vi "Write Receiver.vi"(10 "Receiver":string, 11 "Debug Data In":refnum<class "Debug Data.lvclass">) -> (3 "Debug Data Out":refnum<class "Debug Data.lvclass">)   [LabVIEW 2020, in "Debug Data.lvclass"]
uses:
  Debug Data.lvclass
  Debug Data.lvclass/Debug Data.ctl
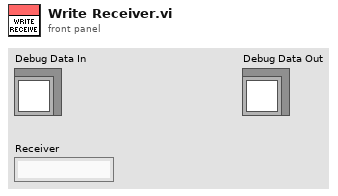
[diagram p1: front panel]
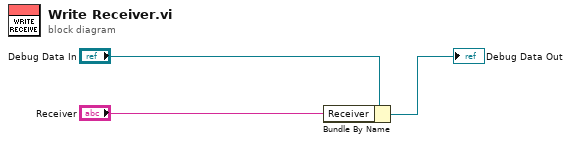
[diagram p0: block diagram]
diagram:
  n1 = Bundle By Name(cluster="Debug Data In", "Receiver"="Receiver") -> (→"Debug Data Out":refnum<class "Debug Data.lvclass">)
